vi "overTempTest.vi"() -> ()   [LabVIEW 2021]
panel:
  in  "-Channel":u16
  in  "+Channel":u16
  in  "Channel":u16
  out "Error Message":string
  out "Temperature (Deg C)":dbl format="%.2f"
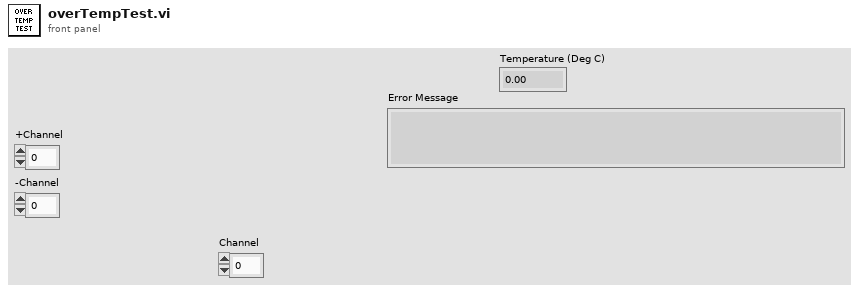
[diagram p1: front panel]
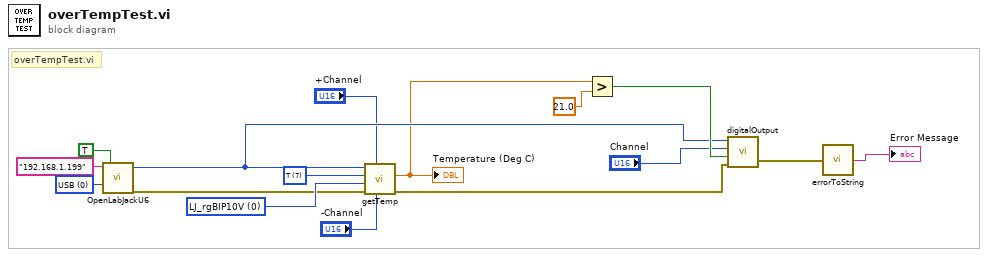
[diagram p0: block diagram]
diagram:
  w12 = u16 0 items=["LJ_rgBIP10V", "LJ_rgBIP5V", "LJ_rgUNI5V", "LJ_rgUNI2P5V", "LJ_rgUNI1P25V", "LJ_rgBIP1V", "LJ_rgUNIP625V", "LJ_rgBIPP1V", "LJ_rgBIPP01V"] ("AIN Range")
  w13 = u16 7 items=["B", "E", "J", "K", "N", "R", "S", "T"] ("Thermocouple Type")
  w15 = u16 0 items=["USB", "Ethernet"] ("Connection Type")
  # "overTempTest.vi"
  n1 = call "OpenLabJackU6.vi"("Select First Found"=TRUE, "Connection Type"=w15, "U6 Address"="192.168.1.199") -> ("error out"=w11:errorcluster, "Handle"=w7:i32)  [unwired: 1 in, 1 out]
  n2 = call "getTemp.vi"("-Channel"="-Channel", "+Channel"="+Channel", "error in"=w11, "AIN Range"=w12, "Thermocouple Type"=w13, "Handle In"=w7) -> ("error out"=w10:errorcluster, "Temperature (Deg C)"=w6:dbl)  [unwired: 1 in, 3 out]
  "Temperature (Deg C)" <- w6
  n3 = Greater?(x=w6, y=21.0) -> (0:w8:bool)
  n4 = call "digitalOutput.vi"("error in"=w10, "State"=w8, "Channel"="Channel", "Handle In"=w7) -> ("error out"=w5:errorcluster)  [unwired: 1 out]
  n5 = call "errorToString.vi"("error in"=w5) -> ("Error Message"=→"Error Message":string)
